vi "Cluster Bundler Get Typedef Terminal.vi"(8 "error in (no error)":errorcluster, 11 "GObject in":refnum<vi>) -> (0 "error out":errorcluster, 3 "Terminal out":refnum<vi>)   [LabVIEW 2014]
doc: "Returns reference to Terminal where has to be connected Cluster which specify how to Bundle items."
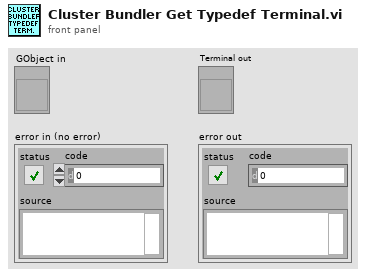
[diagram p1: front panel]
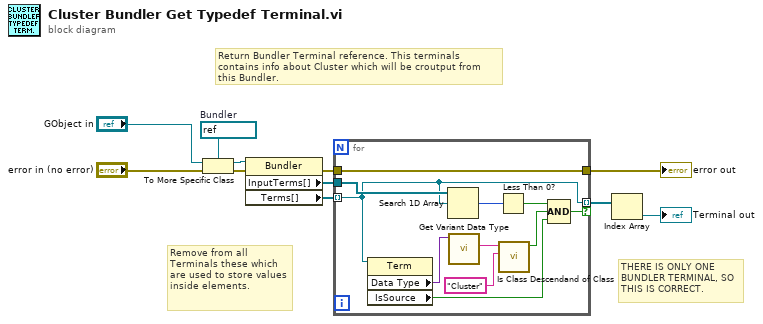
[diagram p0: block diagram]
diagram:
  w2 = refnum<vi> refnum  # Bundler
  # "THERE IS ONLY ONE BUNDLER TERMINAL, SO THIS IS CORRECT."
  # "Remove from all Terminals these which are used to store values inside elements."
  # "Return Bundler Terminal reference. This terminals contains info about Cluster which will be croutput from this Bundler."
  n1 = To More Specific Class(target class=w2, reference="GObject in", error in="error in (no error)") -> (specific class reference=w3:refnum<vi>, error out=w4:errorcluster)
  n2 = property on="Property Node" class="Bundler"(reference=w3, error in=w4) -> (error out=w10:errorcluster, "InputTerms[]"=w6:refnum<vi>[], "Terms[]"=w5:refnum<vi>[])  [unwired: 1 out]
  n3 = for {
    tunnel: w5 -> [w18] mode=indexing
    tunnel: w6 -> [w22]
    tunnel: [w18] -> w7 mode=indexing if=w17
    tunnel: w10 -> [w15]
    tunnel: [w15] -> w11
    n4 = property class="Term"(reference=w18) -> ("Data Type"=w20:variant, "IsSource"=w16:bool)  [unwired: 1 in, 2 out]
    n5 = Search 1D Array(1D array=w22, element=w18) -> (index of element=w21:i32)  [unwired: 1 in]
    n6 = call "Get Variant Data Type.vi"("Variant in"=w20) -> ("first data type"=w13:string)  [unwired: 9 in, 1 out]
    n7 = Less Than 0?(x=w21) -> (x < 0?=w19:bool)
    n8 = call "Is Class Descendand of Class.vi"("Parent ClassName"="Cluster" ("x"), "ClassName"=w13) -> ("is Class descendant?"=w12:bool)  [unwired: 8 in, 1 out]
    n9 = Compound Arithmetic op=AND(w19, w12, w16) -> (w17:bool)
  }
  "error out" <- w11
  n10 = Index Array(array=w7) -> (element=→"Terminal out":refnum<vi>)  [unwired: 1 in]
